vi "WebView2 Viewer.vi"(2 "ProjectRef":refnum<vi>, 4 "Extra Scripts":string, 5 "FileDependency In":map{path, T1}(c390), 6 "Options":string, 7 "OpenWebBrowser(False)":bool, 8 "error in":errorcluster, 9 "Embedd VISJS Librarya in HTMl File(False)":bool, 10 "HTMLFilePath":path, 11 "LibraryDependency":map{path, T3}(c390)) -> (0 "error out":errorcluster, 3 "HTMLFileContent":string)   [LabVIEW 2020, in "WebView2-Viewer.lvlib"] (continued)
OC9OHaTidieicb9ouVAhKtouAseI710ma7pLuqwmgYfHqAFt+6WdLoQ/LBl11Lm7VudAa8vb72PCin9TlAWIsGGhLACD+kSAZnusYBii1XQAPYWDllt6ov2lrBkDBR2+6Ofuak2//3M+G/T4wAAPW7fPhKfRTVeqk9qQbFKRmDUTxS3N7QYGYmwzCkqklBGlPDEcTNv+sg9tNCbTXuvBWujE0bHrZj9JE1B/wU1Pm5PwJN6YBS9a2kVvQEcWnrh5GTFD3lxkYkqRMgYQlwVldUvDnen73LHTUuqitdKM0eAr9AFQfd1J/yo2aJn+2sn4Wdn5qEFODJskgBIjx5T0uCrQA08pnIjS9PERDjPnfOKXAMEBECUoGEIHBj+2zkt76UQ6dXheGAev3+cg74Kf6uJPqcicbfuond7cPy4SOiy7+tD9nFvZurx00KOk3CNEC+mE+vjSPBc7IWqgqTaPT60IMcO/xsXGa3HfKjRgRdbl7/KDg0jtubje6aHj7c7J3dgLQ2zoPwwQ91SooOQdAW1VKVMHty0kA5Bb48BycJn/LjWFGbLv4thvvb53kFvjJ+XEdWkPfjQVR/CcNKYgGMc8JWt5Fa2j+MIPPuyI2pa4IoHSkt6vLIuRaQ9q32khzt4GCxtNu6k46GeiIR2lIfDQQsafPzq1LGRGL9Gk9d+vrwewvfHPQOoexQVjxdB/auk/zmaUMdsfz6bVUtIalT7bxveP1ZHh6GPDPYeSzeD69kcpIfxymFWLNrka+ljhBTWkWwz2JiJT84YHnz2iPx0P20PkmRF5i6HYiwZFJsn/YzdezbzE3cQibY5xV266z6RfXohakb+xB9CjanCD9qTbW7Grk4WV38VZm0l6dhQiEw9taHSuDqrS0FIfDwXM3X9mHMsvRAk/sauDpQy38P+GtzOTGB9mEpkD0C2dS8n8zOjqK9ng8WJZFU+JTjasGvaCNXPpvJBPoMlm0OoDNMfWVxONfWNSUPUZ7TUQ56tCZlPwSgMnJSVRpaSmxsbFE1raw82ZxAZZRQUiBYUKGp5UlOX2krBzmoUVjiIKhHge9rfPo+Wcy3ZeXIYASgL1/X5RfMXMvj46OosrLy7HZbGitUUohIuzoem0RofALaOsghgWGjky0MiJTL8b0lOvI8hN1DKXKP0jd3TNTWDgcJhgMoo4ePYrD4Yi+KmaeLlprnrtXFo9h/AAlG1AqE8yFmBrC+jO0bgH9EVpO/1F2Dc5g//OAsbEx/j0Af+USsQynL1UAAAAASUVORK5CYII=\")}div.vis-network div.vis-edit-mode div.vis-label,div.vis-network div.vis-manipulation div.vis-label{line-height:25px;margin:0 0 0 23px}div.vis-network div.vis-manipulation div.vis-separator-line{background-color:#bdbdbd;display:inline-block;float:left;height:21px;margin:0 7px 0 15px;width:1px}');var jM=function(){function g(t,A,e,C){var I,i,o=this;cn(this,g),this.body=t,this.canvas=A,this.selectionHandler=e,this.interactionHandler=C,this.editMode=!1,this.manipulationDiv=void 0,this.editModeDiv=void 0,this.closeDiv=void 0,this._domEventListenerCleanupQueue=[],this.temporaryUIFunctions={},this.temporaryEventFunctions=[],this.touchTime=0,this.temporaryIds={nodes:[],edges:[]},this.guiEnabled=!1,this.inMode=!1,this.selectedControlNode=void 0,this.options={},this.defaultOptions={enabled:!1,initiallyActive:!1,addNode:!0,addEdge:!0,editNode:void 0,editEdge:!0,deleteNode:!0,deleteEdge:!0,controlNodeStyle:{shape:\"dot\",size:6,color:{background:\"#ff0000\",border:\"#3c3c3c\",highlight:{background:\"#07f968\",border:\"#3c3c3c\"}},borderWidth:2,borderWidthSelected:2}},fe(this.options,this.defaultOptions),this.body.emitter.on(\"destroy\",(function(){o._clean()})),this.body.emitter.on(\"_dataChanged\",je(I=this._restore).call(I,this)),this.body.emitter.on(\"_resetData\",je(i=this._restore).call(i,this))}return kd(g,[{key:\"_restore\",value:function(){!1!==this.inMode&&(!0===this.options.initiallyActive?this.enableEditMode():this.disableEditMode())}},{key:\"setOptions\",value:function(g,t,A){void 0!==t&&(void 0!==t.locale?this.options.locale=t.locale:this.options.locale=A.locale,void 0!==t.locales?this.options.locales=t.locales:this.options.locales=A.locales),void 0!==g&&(\"boolean\"==typeof g?this.options.enabled=g:(this.options.enabled=!0,qf(this.options,g)),!0===this.options.initiallyActive&&(this.editMode=!0),this._setup())}},{key:\"toggleEditMode\",value:function(){!0===this.editMode?this.disableEditMode():this.enableEditMode()}},{key:\"enableEditMode\",value:function(){this.editMode=!0,this._clean(),!0===this.guiEnabled&&(this.manipulationDiv.style.display=\"block\",this.closeDiv.style.display=\"block\",this.editModeDiv.style.display=\"none\",this.showManipulatorToolbar())}},{key:\"disableEditMode\",value:function(){this.editMode=!1,this._clean(),!0===this.guiEnabled&&(this.manipulationDiv.style.display=\"none\",this.closeDiv.style.display=\"none\",this.editModeDiv.style.display=\"block\",this._createEditButton())}},{key:\"showManipulatorToolbar\",value:function(){if(this._clean(),this.manipulationDOM={},!0===this.guiEnabled){var g,t;this.editMode=!0,this.manipulationDiv.style.display=\"block\",this.closeDiv.style.display=\"block\";var A=this.selectionHandler.getSelectedNodeCount(),e=this.selectionHandler.getSelectedEdgeCount(),C=A+e,I=this.options.locales[this.options.locale],i=!1;!1!==this.options.addNode&&(this._createAddNodeButton(I),i=!0),!1!==this.options.addEdge&&(!0===i?this._createSeperator(1):i=!0,this._createAddEdgeButton(I)),1===A&&\"function\"==typeof this.options.editNode?(!0===i?this._createSeperator(2):i=!0,this._createEditNodeButton(I)):1===e&&0===A&&!1!==this.options.editEdge&&(!0===i?this._createSeperator(3):i=!0,this._createEditEdgeButton(I)),0!==C&&(A>0&&!1!==this.options.deleteNode||0===A&&!1!==this.options.deleteEdge)&&(!0===i&&this._createSeperator(4),this._createDeleteButton(I)),this._bindElementEvents(this.closeDiv,je(g=this.toggleEditMode).call(g,this)),this._temporaryBindEvent(\"select\",je(t=this.showManipulatorToolbar).call(t,this))}this.body.emitter.emit(\"_redraw\")}},{key:\"addNodeMode\",value:function(){var g;if(!0!==this.editMode&&this.enableEditMode(),this._clean(),this.inMode=\"addNode\",!0===this.guiEnabled){var t,A=this.options.locales[this.options.locale];this.manipulationDOM={},this._createBackButton(A),this._createSeperator(),this._createDescription(A.addDescription||this.options.locales.en.addDescription),this._bindElementEvents(this.closeDiv,je(t=this.toggleEditMode).call(t,this))}this._temporaryBindEvent(\"click\",je(g=this._performAddNode).call(g,this))}},{key:\"editNode\",value:function(){var g=this;!0!==this.editMode&&this.enableEditMode(),this._clean();var t=this.selectionHandler.getSelectedNodes()[0];if(void 0!==t){if(this.inMode=\"editNode\",\"function\"!=typeof this.options.editNode)throw new Error(\"No function has been configured to handle the editing of nodes.\");if(!0!==t.isCluster){var A=qf({},t.options,!1);if(A.x=t.x,A.y=t.y,2!==this.options.editNode.length)throw new Error(\"The function for edit does not support two arguments (data, callback)\");this.options.editNode(A,(function(t){null!=t&&\"editNode\"===g.inMode&&g.body.data.nodes.getDataSet().update(t),g.showManipulatorToolbar()}))}else alert(this.options.locales[this.options.locale].editClusterError||this.options.locales.en.editClusterError)}else this.showManipulatorToolbar()}},{key:\"addEdgeMode\",value:function(){var g,t,A,e,C;if(!0!==this.editMode&&this.enableEditMode(),this._clean(),this.inMode=\"addEdge\",!0===this.guiEnabled){var I,i=this.options.locales[this.options.locale];this.manipulationDOM={},this._createBackButton(i),this._createSeperator(),this._createDescription(i.edgeDescription||this.options.locales.en.edgeDescription),this._bindElementEvents(this.closeDiv,je(I=this.toggleEditMode).call(I,this))}this._temporaryBindUI(\"onTouch\",je(g=this._handleConnect).call(g,this)),this._temporaryBindUI(\"onDragEnd\",je(t=this._finishConnect).call(t,this)),this._temporaryBindUI(\"onDrag\",je(A=this._dragControlNode).call(A,this)),this._temporaryBindUI(\"onRelease\",je(e=this._finishConnect).call(e,this)),this._temporaryBindUI(\"onDragStart\",je(C=this._dragStartEdge).call(C,this)),this._temporaryBindUI(\"onHold\",(function(){}))}},{key:\"editEdgeMode\",value:function(){if(!0!==this.editMode&&this.enableEditMode(),this._clean(),this.inMode=\"editEdge\",\"object\"!==yd(this.options.editEdge)||\"function\"!=typeof this.options.editEdge.editWithoutDrag||(this.edgeBeingEditedId=this.selectionHandler.getSelectedEdgeIds()[0],void 0===this.edgeBeingEditedId)){if(!0===this.guiEnabled){var g,t=this.options.locales[this.options.locale];this.manipulationDOM={},this._createBackButton(t),this._createSeperator(),this._createDescription(t.editEdgeDescription||this.options.locales.en.editEdgeDescription),this._bindElementEvents(this.closeDiv,je(g=this.toggleEditMode).call(g,this))}if(this.edgeBeingEditedId=this.selectionHandler.getSelectedEdgeIds()[0],void 0!==this.edgeBeingEditedId){var A,e,C,I,i=this.body.edges[this.edgeBeingEditedId],o=this._getNewTargetNode(i.from.x,i.from.y),n=this._getNewTargetNode(i.to.x,i.to.y);this.temporaryIds.nodes.push(o.id),this.temporaryIds.nodes.push(n.id),this.body.nodes[o.id]=o,this.body.nodeIndices.push(o.id),this.body.nodes[n.id]=n,this.body.nodeIndices.push(n.id),this._temporaryBindUI(\"onTouch\",je(A=this._controlNodeTouch).call(A,this)),this._temporaryBindUI(\"onTap\",(function(){})),this._temporaryBindUI(\"onHold\",(function(){})),this._temporaryBindUI(\"onDragStart\",je(e=this._controlNodeDragStart).call(e,this)),this._temporaryBindUI(\"onDrag\",je(C=this._controlNodeDrag).call(C,this)),this._temporaryBindUI(\"onDragEnd\",je(I=this._controlNodeDragEnd).call(I,this)),this._temporaryBindUI(\"onMouseMove\",(function(){})),this._temporaryBindEvent(\"beforeDrawing\",(function(g){var t=i.edgeType.findBorderPositions(g);!1===o.selected&&(o.x=t.from.x,o.y=t.from.y),!1===n.selected&&(n.x=t.to.x,n.y=t.to.y)})),this.body.emitter.emit(\"_redraw\")}else this.showManipulatorToolbar()}else{var r=this.body.edges[this.edgeBeingEditedId];this._performEditEdge(r.from.id,r.to.id)}}},{key:\"deleteSelected\",value:function(){var g=this;!0!==this.editMode&&this.enableEditMode(),this._clean(),this.inMode=\"delete\";var t=this.selectionHandler.getSelectedNodeIds(),A=this.selectionHandler.getSelectedEdgeIds(),e=void 0;if(t.length>0){for(var C=0;C<t.length;C++)if(!0===this.body.nodes[t[C]].isCluster)return void alert(this.options.locales[this.options.locale].deleteClusterError||this.options.locales.en.deleteClusterError);\"function\"==typeof this.options.deleteNode&&(e=this.options.deleteNode)}else A.length>0&&\"function\"==typeof this.options.deleteEdge&&(e=this.options.deleteEdge);if(\"function\"==typeof e){var I={nodes:t,edges:A};if(2!==e.length)throw new Error(\"The function for delete does not support two arguments (data, callback)\");e(I,(function(t){null!=t&&\"delete\"===g.inMode?(g.body.data.edges.getDataSet().remove(t.edges),g.body.data.nodes.getDataSet().remove(t.nodes),g.body.emitter.emit(\"startSimulation\"),g.showManipulatorToolbar()):(g.body.emitter.emit(\"startSimulation\"),g.showManipulatorToolbar())}))}else this.body.data.edges.getDataSet().remove(A),this.body.data.nodes.getDataSet().remove(t),this.body.emitter.emit(\"startSimulation\"),this.showManipulatorToolbar()}},{key:\"_setup\",value:function(){!0===this.options.enabled?(this.guiEnabled=!0,this._createWrappers(),!1===this.editMode?this._createEditButton():this.showManipulatorToolbar()):(this._removeManipulationDOM(),this.guiEnabled=!1)}},{key:\"_createWrappers\",value:function(){var g,t;(void 0===this.manipulationDiv&&(this.manipulationDiv=document.createElement(\"div\"),this.manipulationDiv.className=\"vis-manipulation\",!0===this.editMode?this.manipulationDiv.style.display=\"block\":this.manipulationDiv.style.display=\"none\",this.canvas.frame.appendChild(this.manipulationDiv)),void 0===this.editModeDiv&&(this.editModeDiv=document.createElement(\"div\"),this.editModeDiv.className=\"vis-edit-mode\",!0===this.editMode?this.editModeDiv.style.display=\"none\":this.editModeDiv.style.display=\"block\",this.canvas.frame.appendChild(this.editModeDiv)),void 0===this.closeDiv)&&(this.closeDiv=document.createElement(\"button\"),this.closeDiv.className=\"vis-close\",this.closeDiv.setAttribute(\"aria-label\",null!==(g=null===(t=this.options.locales[this.options.locale])||void 0===t?void 0:t.close)&&void 0!==g?g:this.options.locales.en.close),this.closeDiv.style.display=this.manipulationDiv.style.display,this.canvas.frame.appendChild(this.closeDiv))}},{key:\"_getNewTargetNode\",value:function(g,t){var A=qf({},this.options.controlNodeStyle);A.id=\"targetNode\"+rD(),A.hidden=!1,A.physics=!1,A.x=g,A.y=t;var e=this.body.functions.createNode(A);return e.shape.boundingBox={left:g,right:g,top:t,bottom:t},e}},{key:\"_createEditButton\",value:function(){var g;this._clean(),this.manipulationDOM={},Qf(this.editModeDiv);var t=this.options.locales[this.options.locale],A=this._createButton(\"editMode\",\"vis-edit vis-edit-mode\",t.edit||this.options.locales.en.edit);this.editModeDiv.appendChild(A),this._bindElementEvents(A,je(g=this.toggleEditMode).call(g,this))}},{key:\"_clean\",value:function(){this.inMode=!1,!0===this.guiEnabled&&(Qf(this.editModeDiv),Qf(this.manipulationDiv),this._cleanupDOMEventListeners()),this._cleanupTemporaryNodesAndEdges(),this._unbindTemporaryUIs(),this._unbindTemporaryEvents(),this.body.emitter.emit(\"restorePhysics\")}},{key:\"_cleanupDOMEventListeners\",value:function(){var g,t,A=FM(Zl(g=this._domEventListenerCleanupQueue).call(g,0));try{for(A.s();!(t=A.n()).done;){(0,t.value)()}}catch(g){A.e(g)}finally{A.f()}}},{key:\"_removeManipulationDOM\",value:function(){this._clean(),Qf(this.manipulationDiv),Qf(this.editModeDiv),Qf(this.closeDiv),this.manipulationDiv&&this.canvas.frame.removeChild(this.manipulationDiv),this.editModeDiv&&this.canvas.frame.removeChild(this.editModeDiv),this.closeDiv&&this.canvas.frame.removeChild(this.closeDiv),this.manipulationDiv=void 0,this.editModeDiv=void 0,this.closeDiv=void 0}},{key:\"_createSeperator\",value:function(){var g=arguments.length>0&&void 0!==arguments[0]?arguments[0]:1;this.manipulationDOM[\"seperatorLineDiv\"+g]=document.createElement(\"div\"),this.manipulationDOM[\"seperatorLineDiv\"+g].className=\"vis-separator-line\",this.manipulationDiv.appendChild(this.manipulationDOM[\"seperatorLineDiv\"+g])}},{key:\"_createAddNodeButton\",value:function(g){var t,A=this._createButton(\"addNode\",\"vis-add\",g.addNode||this.options.locales.en.addNode);this.manipulationDiv.appendChild(A),this._bindElementEvents(A,je(t=this.addNodeMode).call(t,this))}},{key:\"_createAddEdgeButton\",value:function(g){var t,A=this._createButton(\"addEdge\",\"vis-connect\",g.addEdge||this.options.locales.en.addEdge);this.manipulationDiv.appendChild(A),this._bindElementEvents(A,je(t=this.addEdgeMode).call(t,this))}},{key:\"_createEditNodeButton\",value:function(g){var t,A=this._createButton(\"editNode\",\"vis-edit\",g.editNode||this.options.locales.en.editNode);this.manipulationDiv.appendChild(A),this._bindElementEvents(A,je(t=this.editNode).call(t,this))}},{key:\"_createEditEdgeButton\",value:function(g){var t,A=this._createButton(\"editEdge\",\"vis-edit\",g.editEdge||this.options.locales.en.editEdge);this.manipulationDiv.appendChild(A),this._bindElementEvents(A,je(t=this.editEdgeMode).call(t,this))}},{key:\"_createDeleteButton\",value:function(g){var t,A;A=this.options.rtl?\"vis-delete-rtl\":\"vis-delete\";var e=this._createButton(\"delete\",A,g.del||this.options.locales.en.del);this.manipulationDiv.appendChild(e),this._bindElementEvents(e,je(t=this.deleteSelected).call(t,this))}},{key:\"_createBackButton\",value:function(g){var t,A=this._createButton(\"back\",\"vis-back\",g.back||this.options.locales.en.back);this.manipulationDiv.appendChild(A),this._bindElementEvents(A,je(t=this.showManipulatorToolbar).call(t,this))}},{key:\"_createButton\",value:function(g,t,A){var e=arguments.length>3&&void 0!==arguments[3]?arguments[3]:\"vis-label\";return this.manipulationDOM[g+\"Div\"]=document.createElement(\"button\"),this.manipulationDOM[g+\"Div\"].className=\"vis-button \"+t,this.manipulationDOM[g+\"Label\"]=document.createElement(\"div\"),this.manipulationDOM[g+\"Label\"].className=e,this.manipulationDOM[g+\"Label\"].innerText=A,this.manipulationDOM[g+\"Div\"].appendChild(this.manipulationDOM[g+\"Label\"]),this.manipulationDOM[g+\"Div\"]}},{key:\"_createDescription\",value:function(g){this.manipulationDOM.descriptionLabel=document.createElement(\"div\"),this.manipulationDOM.descriptionLabel.className=\"vis-none\",this.manipulationDOM.descriptionLabel.innerText=g,this.manipulationDiv.appendChild(this.manipulationDOM.descriptionLabel)}},{key:\"_temporaryBindEvent\",value:function(g,t){this.temporaryEventFunctions.push({event:g,boundFunction:t}),this.body.emitter.on(g,t)}},{key:\"_temporaryBindUI\",value:function(g,t){if(void 0===this.body.eventListeners[g])throw new Error(\"This UI function does not exist. Typo? You tried: \"+g+\" possible are: \"+eu(Lh(this.body.eventListeners)));this.temporaryUIFunctions[g]=this.body.eventListeners[g],this.body.eventListeners[g]=t}},{key:\"_unbindTemporaryUIs\",value:function(){for(var g in this.temporaryUIFunctions)Object.prototype.hasOwnProperty.call(this.temporaryUIFunctions,g)&&(this.body.eventListeners[g]=this.temporaryUIFunctions[g],delete this.temporaryUIFunctions[g]);this.temporaryUIFunctions={}}},{key:\"_unbindTemporaryEvents\",value:function(){for(var g=0;g<this.temporaryEventFunctions.length;g++){var t=this.temporaryEventFunctions[g].event,A=this.temporaryEventFunctions[g].boundFunction;this.body.emitter.off(t,A)}this.temporaryEventFunctions=[]}},{key:\"_bindElementEvents\",value:function(g,t){var A=new Ev(g,{});AP(A,t),this._domEventListenerCleanupQueue.push((function(){A.destroy()}));var e=function(g){var A=g.keyCode,e=g.key;\"Enter\"!==e&&\" \"!==e&&13!==A&&32!==A||t()};g.addEventListener(\"keyup\",e,!1),this._domEventListenerCleanupQueue.push((function(){g.removeEventListener(\"keyup\",e,!1)}))}},{key:\"_cleanupTemporaryNodesAndEdges\",value:function(){for(var g=0;g<this.temporaryIds.edges.length;g++){var t;this.body.edges[this.temporaryIds.edges[g]].disconnect(),delete this.body.edges[this.temporaryIds.edges[g]];var A,e=Xc(t=this.body.edgeIndices).call(t,this.temporaryIds.edges[g]);if(-1!==e)Zl(A=this.body.edgeIndices).call(A,e,1)}for(var C=0;C<this.temporaryIds.nodes.length;C++){var I;delete this.body.nodes[this.temporaryIds.nodes[C]];var i,o=Xc(I=this.body.nodeIndices).call(I,this.temporaryIds.nodes[C]);if(-1!==o)Zl(i=this.body.nodeIndices).call(i,o,1)}this.temporaryIds={nodes:[],edges:[]}}},{key:\"_controlNodeTouch\",value:function(g){this.selectionHandler.unselectAll(),this.lastTouch=this.body.functions.getPointer(g.center),this.lastTouch.translation=fe({},this.body.view.translation)}},{key:\"_controlNodeDragStart\",value:function(){var g=this.lastTouch,t=this.selectionHandler._pointerToPositionObject(g),A=this.body.nodes[this.temporaryIds.nodes[0]],e=this.body.nodes[this.temporaryIds.nodes[1]],C=this.body.edges[this.edgeBeingEditedId];this.selectedControlNode=void 0;var I=A.isOverlappingWith(t),i=e.isOverlappingWith(t);!0===I?(this.selectedControlNode=A,C.edgeType.from=A):!0===i&&(this.selectedControlNode=e,C.edgeType.to=e),void 0!==this.selectedControlNode&&this.selectionHandler.selectObject(this.selectedControlNode),this.body.emitter.emit(\"_redraw\")}},{key:\"_controlNodeDrag\",value:function(g){this.body.emitter.emit(\"disablePhysics\");var t=this.body.functions.getPointer(g.center),A=this.canvas.DOMtoCanvas(t);void 0!==this.selectedControlNode?(this.selectedControlNode.x=A.x,this.selectedControlNode.y=A.y):this.interactionHandler.onDrag(g),this.body.emitter.emit(\"_redraw\")}},{key:\"_controlNodeDragEnd\",value:function(g){var t=this.body.functions.getPointer(g.center),A=this.selectionHandler._pointerToPositionObject(t),e=this.body.edges[this.edgeBeingEditedId];if(void 0!==this.selectedControlNode){this.selectionHandler.unselectAll();for(var C=this.selectionHandler._getAllNodesOverlappingWith(A),I=void 0,i=C.length-1;i>=0;i--)if(C[i]!==this.selectedControlNode.id){I=this.body.nodes[C[i]];break}if(void 0!==I&&void 0!==this.selectedControlNode)if(!0===I.isCluster)alert(this.options.locales[this.options.locale].createEdgeError||this.options.locales.en.createEdgeError);else{var o=this.body.nodes[this.temporaryIds.nodes[0]];this.selectedControlNode.id===o.id?this._performEditEdge(I.id,e.to.id):this._performEditEdge(e.from.id,I.id)}else e.updateEdgeType(),this.body.emitter.emit(\"restorePhysics\");this.body.emitter.emit(\"_redraw\")}}},{key:\"_handleConnect\",value:function(g){if((new Date).valueOf()-this.touchTime>100){this.lastTouch=this.body.functions.getPointer(g.center),this.lastTouch.translation=fe({},this.body.view.translation),this.interactionHandler.drag.pointer=this.lastTouch,this.interactionHandler.drag.translation=this.lastTouch.translation;var t=this.lastTouch,A=this.selectionHandler.getNodeAt(t);if(void 0!==A)if(!0===A.isCluster)alert(this.options.locales[this.options.locale].createEdgeError||this.options.locales.en.createEdgeError);
